vi "Run Step.vi"(8 "error in (no error)":errorcluster, 9 "Pause":bool, 10 "Reset":bool, 11 "FormulaG App in":refnum<class "FormulaG App.lvclass">) -> (0 "error out":errorcluster, 2 "Step Results":T1 {"Last Lap" format="%<%M:%S%3u>t"; "Current Lap" format="%<%M:%S%3u>t"}, 3 "FormulaG App out":refnum<class "FormulaG App.lvclass">, 5 "Chart":sgl[][](array[numeric]), 7 "XY Graph":cluster{dbl[], dbl[]}[](array[cluster]))   [LabVIEW 2020, in "FormulaG.lvlib" / "FormulaG App.lvclass"]
uses:
  FormulaG App.lvclass
  FormulaG App.lvclass/FormulaG App.ctl
  FormulaG API/FormulaG API.lvclass
  Step Result.ctl
  1a97511e-9ff5-4edc-9d5a-0ccfa5af8f59.vi
  a78ea4cc-533d-43ce-a781-8183728e7a63.vi
  01a92202-1c60-46ae-987e-cc3b459b4283.vi
  75fc383f-a2c3-47c1-ae49-b65045ae0360.vi
  c150b076-3f5d-44f4-b69f-d951e1430b90.vi
  152a9b09-e8e6-45cd-9b8f-94e93ff36e8e.vi
  5b87792b-5518-4c60-ac18-c9521ed42ae4.vi
panel:
  out "Overall":dbl format="%.6f"
  out "Time":dbl format="%.6f"
  out "Control":dbl format="%.6f"
  out "Info":dbl format="%.6f"
  out "Ranges":dbl format="%.6f"
  out "API Init":dbl format="%.6f"
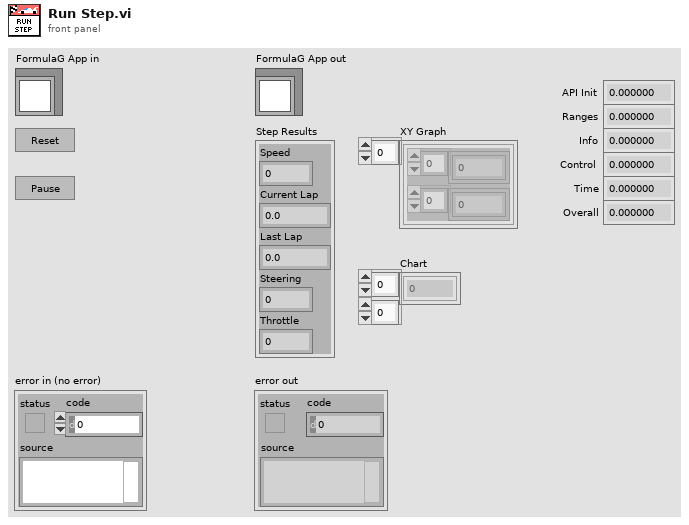
[diagram p1: front panel]
types:
  T1 = typedef "FormulaG.lvlib/FormulaG App.lvclass/Step Result.ctl" = cluster{"Speed":sgl, "Current Lap":dbl, "Last Lap":dbl, "Steering":sgl, "Throttle":sgl}
  T2 = typedef "FormulaG-Common.lvlib/Control VI.ctl" = refnum<vi>
  T3 = typedef "FormulaG-Common.lvlib/Ranges.ctl" = cluster{"Front":sgl[], "Rear":sgl[]}
  T4 = typedef "FormulaG-Common.lvlib/Car State.ctl" = cluster{"Ranges":T3, "Car Info":T5, "Current Lap":dbl, "Last Lap":dbl}
  T5 = typedef "FormulaG-Common.lvlib/Car Info.ctl" = cluster{"Speed":sgl, "X":sgl, "Y":sgl, "Heading":sgl}
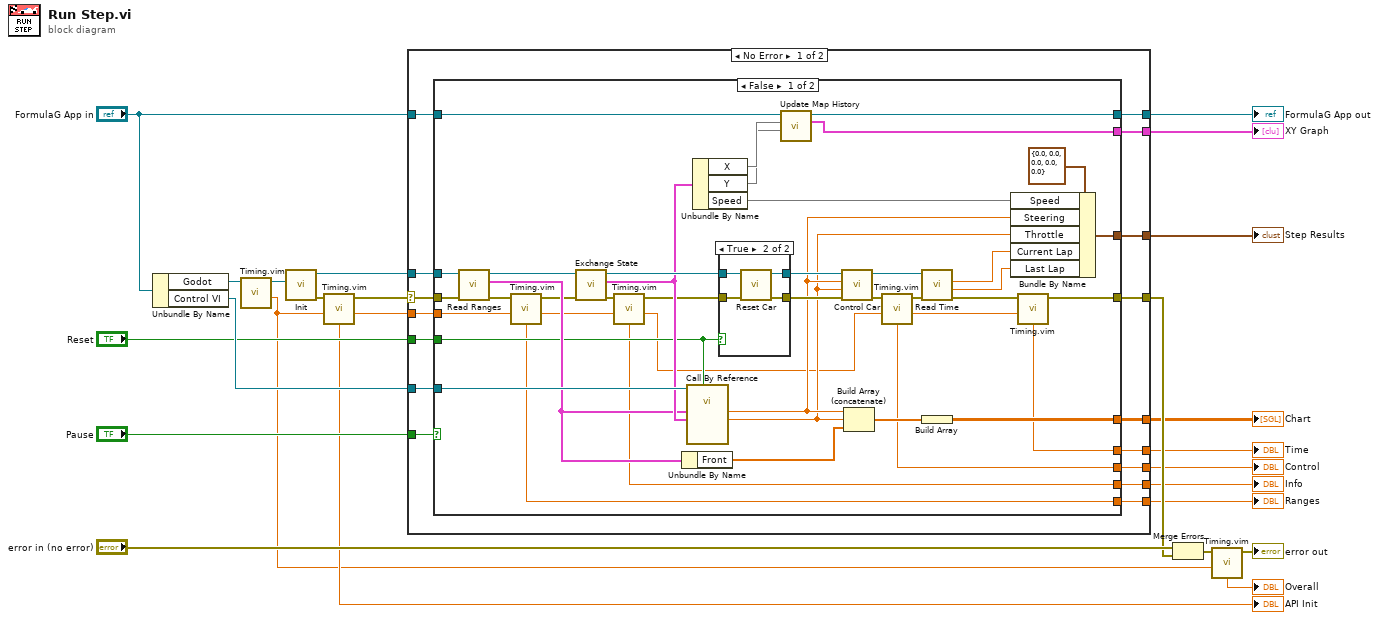
[diagram p0: block diagram]
diagram:
  n1 = Unbundle By Name("FormulaG App in") -> ("Godot"=w23:refnum<class "GodotServer.lvclass">, "Control VI"=w24:T2)
  n2 = call "Timing.vim"("Wire in"=w23) -> ("Now"=w2:dbl, "Wire"=w11:refnum<class "GodotServer.lvclass">)  [unwired: 7 in, 1 out]
  n3 = call "Init.vi"("Godot"=w11) -> ("error out"=w21:errorcluster, "FormulaG API out"=w22:refnum<class "FormulaG API.lvclass">)  [unwired: 9 in]
  n4 = call "Timing.vim"("Previous"=w2, "Wire in"=w21) -> ("Delta"=→"API Init":dbl, "Now"=w8:dbl, "Wire"=w10:errorcluster)  [unwired: 6 in]
  n5 = case shown="No Error" w10 {
    selector: w10 -> [w39 w92]
    tunnel: w22 -> [w41 _]
    tunnel: w24 -> [w40 _]
    tunnel: "FormulaG App in" -> [w38 w93]
    tunnel: [w37 w93] -> w19
    tunnel: [w36 _] -> w12
    tunnel: "Reset" -> [w35 _]
    tunnel: [w34 _] -> w13
    tunnel: "Pause" -> [w33 _]
    tunnel: [w32 w92] -> w15
    tunnel: [w31 _] -> w14
    tunnel: w8 -> [w30 _]
    tunnel: [w29 _] -> w7
    tunnel: [w28 _] -> w6
    tunnel: [w27 _] -> w5
    tunnel: [w26 _] -> w4
    frame No Error {
      n6 = case shown="False" w33 {
        tunnel: w41 -> [w83 _]
        tunnel: w40 -> [w82 _]
        tunnel: w39 -> [w81 w91]
        tunnel: w38 -> [w68 w90]
        tunnel: [w65 w90] -> w37
        tunnel: [w64 _] -> w36
        tunnel: w35 -> [w63 _]
        tunnel: [w62 _] -> w34
        tunnel: [w48 w91] -> w32
        tunnel: [w54 _] -> w31
        tunnel: w30 -> [w52 _]
        tunnel: [w45 _] -> w29
        tunnel: [w44 _] -> w28
        tunnel: [w43 _] -> w27
        tunnel: [w42 _] -> w26
        frame False {
          n7 = call "Read Ranges.vi"("error in (no error)"=w81, "FormulaG API in"=w83) -> ("error out"=w76:errorcluster, "Ranges"=w72:T3, "FormulaG API out"=w75:refnum<class "FormulaG API.lvclass">)  [unwired: 7 in]
          n8 = call "Timing.vim"("Previous"=w52, "Wire in"=w76) -> ("Delta"=w45:dbl, "Now"=w50:dbl, "Wire"=w53:errorcluster)  [unwired: 6 in]
          n9 = call "Exchange State.vi"("error in (no error)"=w53, "FormulaG API in"=w75) -> ("error out"=w78:errorcluster, "Car State"=w73:T4, "FormulaG API out"=w74:refnum<class "FormulaG API.lvclass">)  [unwired: 7 in]
          n10 = call "Timing.vim"("Previous"=w50, "Wire in"=w78) -> ("Delta"=w44:dbl, "Now"=w46:dbl, "Wire"=w51:errorcluster)  [unwired: 6 in]
          n11 = Unbundle By Name(w72) -> ("Front"=w71:sgl[])
          n12 = call-by-ref "?"(reference=w82, "Reset"=w63, "Car Info"=w73, "Ranges"=w72) -> ("Throttle (0 to 1)"=w58:sgl, "Steering (-1 to 1)"=w59:sgl)  [unwired: 8 in, 2 out]
          n13 = Unbundle By Name(w73) -> ("X"=w67, "Y"=w66, "Speed"=w60)
          n14 = case shown="True" w63 {
            tunnel: w74 -> [w85 w89]
            tunnel: [w85 w88] -> w69
            tunnel: w51 -> [w84 w87]
            tunnel: [w84 w86] -> w77
            frame False {
            }
            frame True {
              n15 = call "Reset Car.vi"("error in (no error)"=w87, "FormulaG API in"=w89) -> ("error out"=w86:errorcluster, "FormulaG API out"=w88:refnum<class "FormulaG API.lvclass">)  [unwired: 8 in]
            }
          }
          n16 = call "Update Map History.vi"("Y"=w66, "X"=w67, "FormulaG App in"=w68) -> ("XY Graph"=w64:cluster{dbl[], dbl[]}[], "FormulaG App out"=w65:refnum<class "FormulaG App.lvclass">)  [unwired: 6 in, 1 out]
          n17 = call "Control Car.vi"("error in (no error)"=w77, "Throttle"=w58, "Steering"=w59, "FormulaG API in"=w69) -> ("error out"=w79:errorcluster, "FormulaG API out"=w80:refnum<class "FormulaG API.lvclass">)  [unwired: 6 in]
          n18 = Build Array (concatenate)(w59, w58, w71) -> (w70:sgl[])
          n19 = call "Timing.vim"("Previous"=w46, "Wire in"=w79) -> ("Delta"=w43:dbl, "Now"=w47:dbl, "Wire"=w49:errorcluster)  [unwired: 6 in]
          n20 = call "Read Time.vi"("error in (no error)"=w49, "FormulaG API in"=w80) -> ("error out"=w55:errorcluster, "Last Lap"=w56:dbl, "Current Lap"=w57:dbl)  [unwired: 6 in, 1 out]
          n21 = Build Array(w70) -> (w62:sgl[][])
          n22 = Bundle By Name(cluster=T1 {"Speed"=0.0, "Current Lap"=0.0, "Last Lap"=0.0, "Steering"=0.0, "Throttle"=0.0} ("Step Results"), "Speed"=w60, "Steering"=w59, "Throttle"=w58, "Current Lap"=w57, "Last Lap"=w56) -> (w54:T1)
          n23 = call "Timing.vim"("Previous"=w47, "Wire in"=w55) -> ("Delta"=w42:dbl, "Wire"=w48:errorcluster)  [unwired: 6 in, 1 out]
        }
        frame True {
        }
      }
    }
    frame Error {
    }
  }
  "FormulaG App out" <- w19
  "Step Results" <- w14
  "Chart" <- w13
  "XY Graph" <- w12
  "Ranges" <- w7
  "Info" <- w6
  "Control" <- w5
  "Time" <- w4
  n24 = Merge Errors("error in (no error)", w15) -> (w16:errorcluster)
  n25 = call "Timing.vim"("Previous"=w2, "Wire in"=w16) -> ("Delta"=→"Overall":dbl, "Wire"=→"error out":errorcluster)  [unwired: 6 in, 1 out]
